vi "FlatToRichnixnet_grpc_DeviceRefArray.vi"(5 "OutputClusterType":T1, 11 "InputCluster":T3) -> (3 "OutputCluster":T1)   [LabVIEW 2025, in "xnet-grpc_client.lvlib"]
uses:
  xnet-grpc_client.lvlib
  nixnet_grpc_DeviceRefArray_Flat.ctl
  nidevice_grpc_Session_Flat.ctl
  nixnet_grpc_DeviceRefArray.ctl
  nidevice_grpc_Session.ctl
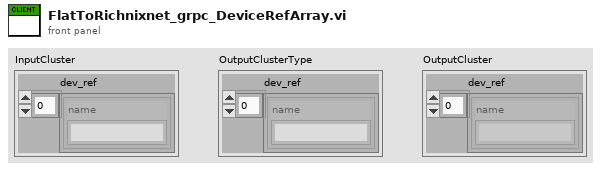
[diagram p1: front panel]
types:
  T1 = typedef "xnet-grpc_client.lvlib/nixnet_grpc_DeviceRefArray.ctl" = cluster{"dev_ref":T2[]}
  T2 = typedef "xnet-grpc_client.lvlib/nidevice_grpc_Session.ctl" = cluster{"name":string}
  T3 = typedef "xnet-grpc_client.lvlib/nixnet_grpc_DeviceRefArray_Flat.ctl" = cluster{"dev_ref":T4[]}
  T4 = typedef "xnet-grpc_client.lvlib/nidevice_grpc_Session_Flat.ctl" = cluster{"name":string}
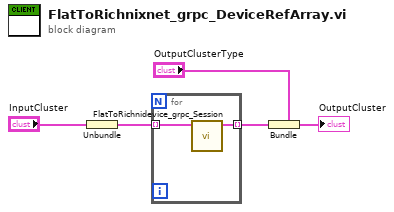
[diagram p0: block diagram]
diagram:
  n1 = Unbundle "Unbundle"("InputCluster") -> ("dev_ref"=w2:T4[])
  n2 = for {
    tunnel: w2 -> [w7] mode=indexing
    tunnel: [w6] -> w1 mode=indexing
    n3 = call "FlatToRichnidevice_grpc_Session.vi"("InputCluster"=w7) -> ("OutputCluster"=w6:T2)  [unwired: 10 in]
  }
  n4 = Bundle "Bundle"(cluster="OutputClusterType", "dev_ref"=w1) -> (→"OutputCluster":T1)
